vi "SimpleStimulation.vi"   [LabVIEW 2017]
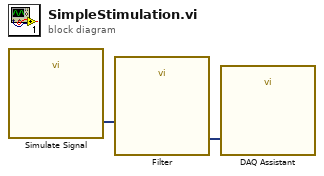
[diagram p0: block diagram]
diagram:
  n1 = call "Simulate Signal"() -> ("DC with Gaussian Noise"=w2:dynamicdata)  [unwired: 14 in, 1 out]
  n2 = call "Filter"("Signal"=w2) -> ("Filtered Signal"=w1:dynamicdata)  [unwired: 9 in, 1 out]
  n3 = call "DAQ Assistant"("data"=w1) -> ()  [unwired: 17 in, 2 out]
